vi "Periodic Tasks.vi"(8 "error in":errorcluster, 11 "Begin Cluster":T2={"Left Drive Encoder"={"DevStatus"={"status"=FALSE, "code"=0, "source"=""}, "EncoderIndex"=enum."Enc 0", "CounterIndex"=enum."Invalid", "DistancePerCount"=1.0, "Decoding Type"=enum."4x"}, "Right Drive Encoder"={"DevStatus"={"status"=FALSE, "code"=0, "source"=""}, "EncoderIndex"=enum."Enc 1", "CounterIndex"=enum."Invalid", "DistancePerCount"=1.0, "Decoding Type"=enum."4x"}, "Elevator Encoder"={"DevStatus"={"status"=FALSE, "code"=0, "source"=""}, "EncoderIndex"=enum."Enc 2", "CounterIndex"=enum."Invalid", "DistancePerCount"=1.0, "Decoding Type"=enum."4x"}, "Drive Shifter"={"DevStatus"={"status"=FALSE, "code"=0, "source"=""}, "Pneumatics Control Module"=0, "Forward Solenoid Channel"=enum."Solenoid 0", "Reverse Solenoid Channel"=enum."Solenoid 1"}, "Elevator Shifter"={"DevStatus"={"status"=FALSE, "code"=0, "source"=""}, "Pneumatics Control Module"=0, "Forward Solenoid Channel"=enum."Solenoid 2", "Reverse Solenoid Channel"=enum."Solenoid 3"}, "Elevator Brake"={"DevStatus"={"status"=FALSE, "code"=0, "source"=""}, "Pneumatics Control Module"=0, "Forward Solenoid Channel"=enum."Solenoid 4", "Reverse Solenoid Channel"=enum."Solenoid 5"}, "Intake Clamp"={"DevStatus"={"status"=FALSE, "code"=0, "source"=""}, "Pneumatics Control Module"=0, "Forward Solenoid Channel"=enum."Invalid", "Reverse Solenoid Channel"=enum."Invalid"}, "Intake Hinge"={"DevStatus"={"status"=FALSE, "code"=0, "source"=""}, "Pneumatics Control Module"=0, "Forward Solenoid Channel"=enum."Invalid", "Reverse Solenoid Channel"=enum."Invalid"}, "Pot Left"={"DevStatus"={"status"=FALSE, "code"=0, "source"=""}, "Analog Channel"=enum."AI 0", "Invert Output"=FALSE}, "Pot Right"={"DevStatus"={"status"=FALSE, "code"=0, "source"=""}, "Analog Channel"=enum."AI 1", "Invert Output"=FALSE}, "Gyro"={"DevStatus"={"status"=FALSE, "code"=0, "source"=""}, "Analog Channel"=enum."AI 1", "Gain (VoltsPerDegree/Second)"=0.0, "Gyro Type"=enum."XRS450", "Handle"=8, "SPI Bus"=enum."SPI On-Board, CS0", "Device Found"=TRUE, "Sample Rate"=2000.0, "Calibrate On Open"=FALSE, "Offset"=0.849940624999998}, "Drive Motors"={"DevStatus"={"status"=FALSE, "code"=0, "source"=""}, "Motors[]"=[{"DeviceStatus"={"status"=FALSE, "code"=0, "source"=""}, "Type"=enum."CAN", "PWM"={"PWM Channel"=enum."PWM 1", "DeadBand"={"Name"="", "maxPositivePwm"=0, "minPositivePwm"=0, "centerPwm"=0, "maxNegativePwm"=0, "minNegativePwm"=0, "angularRange"=0}}, "CAN"={"Device Number"=1, "SetOutput VI Ref"=variant(refnum<vi> refnum), "GetOutput VI Ref"=variant(refnum<vi> refnum), "Enable VI Ref"=variant(refnum<vi> refnum), "Disable VI Ref"=variant(refnum<vi> refnum), "Data"=variant(cluster{"Library":path, "handle":u64, "Control Mode":u16, "UsageFrame":u32, "RefNumName":string, "arbID":u32} {"Library"=path "libCTRE_PhoenixCCI.so", "handle"=38411456, "Control Mode"=0, "UsageFrame"=0, "RefNumName"="", "arbID"=33816577})}, "Invert"=TRUE, "DIO PWM"={"PWM \"Enable\" Channel"=enum."Invalid", "DIOChannel"=enum."Invalid", "PWM Rate"=0.0}}, {"DeviceStatus"={"status"=FALSE, "code"=0, "source"=""}, "Type"=enum."CAN", "PWM"={"PWM Channel"=enum."PWM 1", "DeadBand"={"Name"="", "maxPositivePwm"=0, "minPositivePwm"=0, "centerPwm"=0, "maxNegativePwm"=0, "minNegativePwm"=0, "angularRange"=0}}, "CAN"={"Device Number"=13, "SetOutput VI Ref"=variant(refnum<vi> refnum), "GetOutput VI Ref"=variant(refnum<vi> refnum), "Enable VI Ref"=variant(refnum<vi> refnum), "Disable VI Ref"=variant(refnum<vi> refnum), "Data"=variant(cluster{"Library":path, "handle":u64, "Control Mode":u16, "UsageFrame":u32, "RefNumName":string, "arbID":u32} {"Library"=path "libCTRE_PhoenixCCI.so", "handle"=38441312, "Control Mode"=0, "UsageFrame"=0, "RefNumName"="", "arbID"=33816589})}, "Invert"=FALSE, "DIO PWM"={"PWM \"Enable\" Channel"=enum."Invalid", "DIOChannel"=enum."Invalid", "PWM Rate"=0.0}}], "Square Inputs"=FALSE, "Max Output"=1.0}, "Elevator Master"={"DeviceStatus"={"status"=FALSE, "code"=0, "source"=""}, "Type"=enum."CAN", "PWM"={"PWM Channel"=enum."PWM 1", "DeadBand"={"Name"="", "maxPositivePwm"=0, "minPositivePwm"=0, "centerPwm"=0, "maxNegativePwm"=0, "minNegativePwm"=0, "angularRange"=0}}, "CAN"={"Device Number"=9, "SetOutput VI Ref"=variant(refnum<vi> refnum), "GetOutput VI Ref"=variant(refnum<vi> refnum), "Enable VI Ref"=variant(refnum<vi> refnum), "Disable VI Ref"=variant(refnum<vi> refnum), "Data"=variant(cluster{"Library":path, "handle":u64, "Control Mode":u16, "UsageFrame":u32, "RefNumName":string, "arbID":u32} {"Library"=path "libCTRE_PhoenixCCI.so", "handle"=38410640, "Control Mode"=0, "UsageFrame"=0, "RefNumName"="", "arbID"=33816585})}, "Invert"=TRUE, "DIO PWM"={"PWM \"Enable\" Channel"=enum."Invalid", "DIOChannel"=enum."Invalid", "PWM Rate"=0.0}}, "Intake Left"={"DeviceStatus"={"status"=FALSE, "code"=0, "source"=""}, "Type"=enum."CAN", "PWM"={"PWM Channel"=enum."PWM 1", "DeadBand"={"Name"="", "maxPositivePwm"=0, "minPositivePwm"=0, "centerPwm"=0, "maxNegativePwm"=0, "minNegativePwm"=0, "angularRange"=0}}, "CAN"={"Device Number"=6, "SetOutput VI Ref"=variant(refnum<vi> refnum), "GetOutput VI Ref"=variant(refnum<vi> refnum), "Enable VI Ref"=variant(refnum<vi> refnum), "Disable VI Ref"=variant(refnum<vi> refnum), "Data"=variant(cluster{"Library":path, "handle":u64, "Control Mode":u16, "UsageFrame":u32, "RefNumName":string, "arbID":u32} {"Library"=path "libCTRE_PhoenixCCI.so", "handle"=38393360, "Control Mode"=0, "UsageFrame"=0, "RefNumName"="", "arbID"=33816582})}, "Invert"=FALSE, "DIO PWM"={"PWM \"Enable\" Channel"=enum."Invalid", "DIOChannel"=enum."Invalid", "PWM Rate"=0.0}}, "Intake Right"={"DeviceStatus"={"status"=FALSE, "code"=0, "source"=""}, "Type"=enum."CAN", "PWM"={"PWM Channel"=enum."PWM 1", "DeadBand"={"Name"="", "maxPositivePwm"=0, "minPositivePwm"=0, "centerPwm"=0, "maxNegativePwm"=0, "minNegativePwm"=0, "angularRange"=0}}, "CAN"={"Device Number"=7, "SetOutput VI Ref"=variant(refnum<vi> refnum), "GetOutput VI Ref"=variant(refnum<vi> refnum), "Enable VI Ref"=variant(refnum<vi> refnum), "Disable VI Ref"=variant(refnum<vi> refnum), "Data"=variant(cluster{"Library":path, "handle":u64, "Control Mode":u16, "UsageFrame":u32, "RefNumName":string, "arbID":u32} {"Library"=path "libCTRE_PhoenixCCI.so", "handle"=38392544, "Control Mode"=0, "UsageFrame"=0, "RefNumName"="", "arbID"=33816583})}, "Invert"=FALSE, "DIO PWM"={"PWM \"Enable\" Channel"=enum."Invalid", "DIOChannel"=enum."Invalid", "PWM Rate"=0.0}}, "Linear Actuator Left"={"DeviceStatus"={"status"=FALSE, "code"=0, "source"=""}, "Type"=enum."CAN", "PWM"={"PWM Channel"=enum."PWM 1", "DeadBand"={"Name"="", "maxPositivePwm"=0, "minPositivePwm"=0, "centerPwm"=0, "maxNegativePwm"=0, "minNegativePwm"=0, "angularRange"=0}}, "CAN"={"Device Number"=4, "SetOutput VI Ref"=variant(refnum<vi> refnum), "GetOutput VI Ref"=variant(refnum<vi> refnum), "Enable VI Ref"=variant(refnum<vi> refnum), "Disable VI Ref"=variant(refnum<vi> refnum), "Data"=variant(cluster{"Library":path, "handle":u64, "Control Mode":u16, "UsageFrame":u32, "RefNumName":string, "arbID":u32} {"Library"=path "libCTRE_PhoenixCCI.so", "handle"=36427792, "Control Mode"=0, "UsageFrame"=0, "RefNumName"="", "arbID"=33816580})}, "Invert"=FALSE, "DIO PWM"={"PWM \"Enable\" Channel"=enum."Invalid", "DIOChannel"=enum."Invalid", "PWM Rate"=0.0}}, "Linear Actuator Right"={"DeviceStatus"={"status"=FALSE, "code"=0, "source"=""}, "Type"=enum."CAN", "PWM"={"PWM Channel"=enum."PWM 1", "DeadBand"={"Name"="", "maxPositivePwm"=0, "minPositivePwm"=0, "centerPwm"=0, "maxNegativePwm"=0, "minNegativePwm"=0, "angularRange"=0}}, "CAN"={"Device Number"=5, "SetOutput VI Ref"=variant(refnum<vi> refnum), "GetOutput VI Ref"=variant(refnum<vi> refnum), "Enable VI Ref"=variant(refnum<vi> refnum), "Disable VI Ref"=variant(refnum<vi> refnum), "Data"=variant(cluster{"Library":path, "handle":u64, "Control Mode":u16, "UsageFrame":u32, "RefNumName":string, "arbID":u32} {"Library"=path "libCTRE_PhoenixCCI.so", "handle"=38440496, "Control Mode"=0, "UsageFrame"=0, "RefNumName"="", "arbID"=33816581})}, "Invert"=FALSE, "DIO PWM"={"PWM \"Enable\" Channel"=enum."Invalid", "DIOChannel"=enum."Invalid", "PWM Rate"=0.0}}, "X Joystick"={"Device"=enum."USB 0"}, "Y Joystick"={"Device"=enum."USB 1"}, "Controller"={"Device"=enum."USB 2"}, "775 Drive Motors"={"DevStatus"={"status"=FALSE, "code"=0, "source"=""}, "Motors[]"=[{"DeviceStatus"={"status"=FALSE, "code"=0, "source"=""}, "Type"=enum."CAN", "PWM"={"PWM Channel"=enum."PWM 1", "DeadBand"={"Name"="", "maxPositivePwm"=0, "minPositivePwm"=0, "centerPwm"=0, "maxNegativePwm"=0, "minNegativePwm"=0, "angularRange"=0}}, "CAN"={"Device Number"=3, "SetOutput VI Ref"=variant(refnum<vi> refnum), "GetOutput VI Ref"=variant(refnum<vi> refnum), "Enable VI Ref"=variant(refnum<vi> refnum), "Disable VI Ref"=variant(refnum<vi> refnum), "Data"=variant(cluster{"Library":path, "handle":u64, "Control Mode":u16, "UsageFrame":u32, "RefNumName":string, "arbID":u32} {"Library"=path "libCTRE_PhoenixCCI.so", "handle"=38456632, "Control Mode"=0, "UsageFrame"=0, "RefNumName"="", "arbID"=33816579})}, "Invert"=FALSE, "DIO PWM"={"PWM \"Enable\" Channel"=enum."Invalid", "DIOChannel"=enum."Invalid", "PWM Rate"=0.0}}, {"DeviceStatus"={"status"=FALSE, "code"=0, "source"=""}, "Type"=enum."CAN", "PWM"={"PWM Channel"=enum."PWM 1", "DeadBand"={"Name"="", "maxPositivePwm"=0, "minPositivePwm"=0, "centerPwm"=0, "maxNegativePwm"=0, "minNegativePwm"=0, "angularRange"=0}}, "CAN"={"Device Number"=11, "SetOutput VI Ref"=variant(refnum<vi> refnum), "GetOutput VI Ref"=variant(refnum<vi> refnum), "Enable VI Ref"=variant(refnum<vi> refnum), "Disable VI Ref"=variant(refnum<vi> refnum), "Data"=variant(cluster{"Library":path, "handle":u64, "Control Mode":u16, "UsageFrame":u32, "RefNumName":string, "arbID":u32} {"Library"=path "libCTRE_PhoenixCCI.so", "handle"=36428608, "Control Mode"=0, "UsageFrame"=0, "RefNumName"="", "arbID"=33816587})}, "Invert"=TRUE, "DIO PWM"={"PWM \"Enable\" Channel"=enum."Invalid", "DIOChannel"=enum."Invalid", "PWM Rate"=0.0}}], "Square Inputs"=FALSE, "Max Output"=1.0}, "Intake Angle Encoder"={"DevStatus"={"status"=FALSE, "code"=0, "source"=""}, "EncoderIndex"=enum."Enc 3", "CounterIndex"=enum."Invalid", "DistancePerCount"=1.0, "Decoding Type"=enum."4x"}, "Intake Angle"={"DeviceStatus"={"status"=FALSE, "code"=0, "source"=""}, "Type"=enum."CAN", "PWM"={"PWM Channel"=enum."PWM 1", "DeadBand"={"Name"="", "maxPositivePwm"=0, "minPositivePwm"=0, "centerPwm"=0, "maxNegativePwm"=0, "minNegativePwm"=0, "angularRange"=0}}, "CAN"={"Device Number"=8, "SetOutput VI Ref"=variant(refnum<vi> refnum), "GetOutput VI Ref"=variant(refnum<vi> refnum), "Enable VI Ref"=variant(refnum<vi> refnum), "Disable VI Ref"=variant(refnum<vi> refnum), "Data"=variant(cluster{"Library":path, "handle":u64, "Control Mode":u16, "UsageFrame":u32, "RefNumName":string, "arbID":u32} {"Library"=path "libCTRE_PhoenixCCI.so", "handle"=38391728, "Control Mode"=0, "UsageFrame"=0, "RefNumName"="", "arbID"=33816584})}, "Invert"=FALSE, "DIO PWM"={"PWM \"Enable\" Channel"=enum."Invalid", "DIOChannel"=enum."Invalid", "PWM Rate"=0.0}}} {"Gyro"."Sample Rate" min=0.25 max=100.0 step=0.25}) -> ()   [LabVIEW 2017]
doc: "This VI runs in parallel to other tasks. It can contain as many user-defined periodic loops as you need. These can carry out PID or other sorts of timed response."
uses:
  Begin Cluster.ctl
  <vilib>/Rock Robotics/WPI/Encoder/WPI_EncoderDevRef.ctl
  <vilib>/Rock Robotics/SystemInterfaces/Encoder/FPGA_EncoderIdx.ctl
  <vilib>/Rock Robotics/SystemInterfaces/Counter/FPGA_CounterCtrSystemIndex.ctl
  <vilib>/Rock Robotics/WPI/Encoder/WPI_EncoderType.ctl
  <vilib>/Rock Robotics/WPI/Solenoid/WPI_SolenoidDevRef.ctl
  <vilib>/Rock Robotics/WPI/Solenoid/WPI_SolenoidChannel.ctl
  <vilib>/Rock Robotics/WPI/Potentiometer/WPI_PotentiometerDevRef.ctl
  <vilib>/Rock Robotics/SystemInterfaces/AI/FPGA_AIChannel.ctl
  <vilib>/Rock Robotics/WPI/Gyro/WPI_GyroDevRef.ctl
  <vilib>/Rock Robotics/SystemInterfaces/spilib/spi_bus.ctl
  <vilib>/Rock Robotics/WPI/RobotDrive/WPI_RobotDriveDevRef.ctl
  <vilib>/Rock Robotics/WPI/MotorControl/WPI_MotorControlDeviceRef.ctl
  <vilib>/Rock Robotics/WPI/MotorControl/WPI_MotorControlType.ctl
  <vilib>/Rock Robotics/SystemInterfaces/DIO/FPGA_DIOPWMChannel.ctl
  <vilib>/Rock Robotics/WPI/PWM/WPI_PWMDeadband.ctl
  <vilib>/Rock Robotics/SystemInterfaces/DIO/FPGA_DIOChannel.ctl
  <vilib>/Rock Robotics/WPI/Joystick/WPI_JoystickDevRef.ctl
  <vilib>/Rock Robotics/WPI/Joystick/WPI_JoystickDeviceEnum.ctl
  <vilib>/Rock Robotics/WPI/Solenoid/WPI_SolenoidValue.ctl
  Global Variables.vi
  <vilib>/addons/control/pid/pid.llb/PID (DBL).vi
  <vilib>/Rock Robotics/WPI/Solenoid/WPI_SolenoidSetEnum.vi
  <vilib>/Rock Robotics/Network Tables/NT Read Number.vi
  <vilib>/Rock Robotics/Network Tables/NT Write Boolean.vi
  <vilib>/addons/control/pid/NI_PID_pid.lvlib
panel:
  out "Intake Encoder":dbl
  out "Right Encoder":dbl
  out "Side":dbl
  out "Field option":dbl
  out "Elevator Topped Out":bool
  in  "Intake PID Gains":T1={"proportional gain (Kc)"=0.06610000000000005, "integral time (Ti, min)"=0.0, "derivative time (Td, min)"=0.002} {"derivative time (Td, min)" format="%.3f"; "integral time (Ti, min)" format="%.3f"; "proportional gain (Kc)" format="%.3f"}
  in  "Intake Range":cluster{"output high":dbl, "output low":dbl}={"output high"=1.0, "output low"=-1.0} {"output low" format="%.2f"; "output high" format="%.2f"}
  in  "Elevator Gains High":T1={"proportional gain (Kc)"=0.0008, "integral time (Ti, min)"=0.0, "derivative time (Td, min)"=0.0} {"proportional gain (Kc)" format="%#_7g"}
  out "Elevator Encoder":dbl=-256.25
  out "Normalized Value":dbl=0.6625300700982322
  in  "Elevator Gains Low":T1={"proportional gain (Kc)"=0.0011, "integral time (Ti, min)"=0.0, "derivative time (Td, min)"=0.0} {"derivative time (Td, min)" format="%.3f"; "integral time (Ti, min)" format="%.3f"; "proportional gain (Kc)" format="%.5f"}
  in  "Cube Up":bool
  in  "Cube Down":bool
  out "Angle":dbl=-3.1437039937493667
  out "Left Encoder":dbl=-0.5
  # "Analog"
  # "XRS"
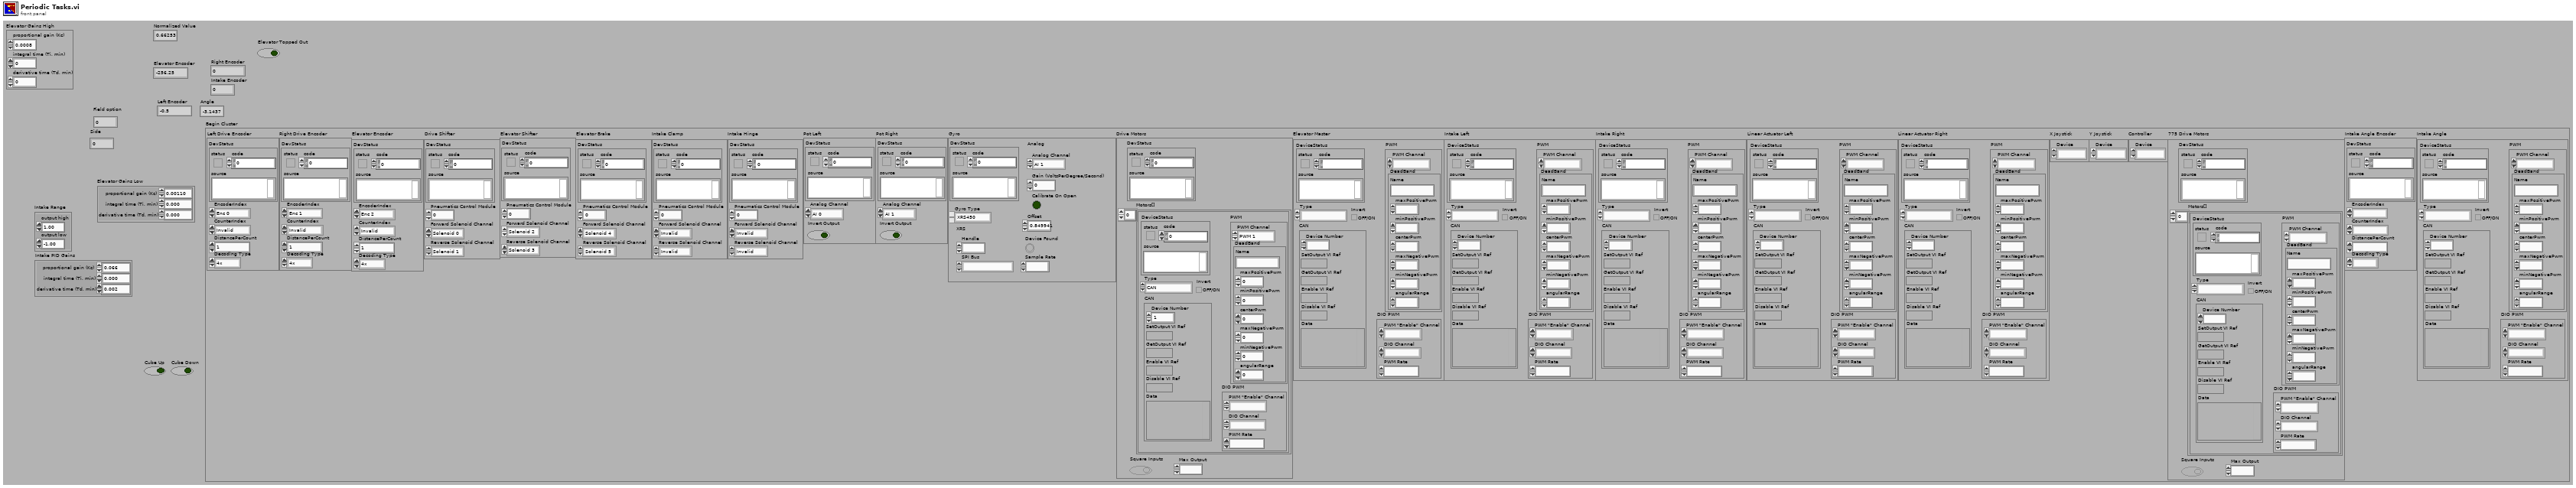
[diagram p1: front panel]
types:
  T1 = cluster{"proportional gain (Kc)":dbl, "integral time (Ti, min)":dbl, "derivative time (Td, min)":dbl}
  T2 = typedef "Begin Cluster.ctl" = cluster{"Left Drive Encoder":T3, "Right Drive Encoder":T3, "Elevator Encoder":T3, "Drive Shifter":T7, "Elevator Shifter":T7, "Elevator Brake":T7, "Intake Clamp":T7, "Intake Hinge":T7, "Pot Left":T9, "Pot Right":T9, "Gyro":T11, "Drive Motors":T13, "Elevator Master":T14, "Intake Left":T14, "Intake Right":T14, "Linear Actuator Left":T14, "Linear Actuator Right":T14, "X Joystick":T19, "Y Joystick":T19, "Controller":T19, "775 Drive Motors":T13, "Intake Angle Encoder":T3, "Intake Angle":T14}
  T3 = typedef "WPI_EncoderDevRef.ctl" = cluster{"DevStatus":errorcluster, "EncoderIndex":T4, "CounterIndex":T5, "DistancePerCount":dbl, "Decoding Type":T6}
  T4 = typedef "FPGA_EncoderIdx.ctl" = enum8{"Enc 0", "Enc 1", "Enc 2", "Enc 3", "Enc 4", "Enc 5", "Enc 6", "Enc 7", "Invalid"}
  T5 = typedef "FPGA_CounterCtrSystemIndex.ctl" = enum8{"Ctr 0", "Ctr 1", "Ctr 2", "Ctr 3", "Ctr 4", "Ctr 5", "Ctr 6", "Ctr 7", "Invalid"}
  T6 = typedef "WPI_EncoderType.ctl" = enum16{"1x", "2x", "4x"}
  T7 = typedef "WPI_SolenoidDevRef.ctl" = cluster{"DevStatus":errorcluster, "Pneumatics Control Module":u8, "Forward Solenoid Channel":T8, "Reverse Solenoid Channel":T8}
  T8 = typedef "WPI_SolenoidChannel.ctl" = enum8{"Solenoid 0", "Solenoid 1", "Solenoid 2", "Solenoid 3", "Solenoid 4", "Solenoid 5", "Solenoid 6", "Solenoid 7", "Invalid"}
  T9 = typedef "WPI_PotentiometerDevRef.ctl" = cluster{"DevStatus":errorcluster, "Analog Channel":T10, "Invert Output":bool}
  T10 = typedef "FPGA_AIChannel.ctl" = enum8{"AI 0", "AI 1", "AI 2", "AI 3", "AI MXP 0", "AI MXP 1", "AI MXP 2", "AI MXP 3", "Invalid"}
  T11 = typedef "WPI_GyroDevRef.ctl" = cluster{"DevStatus":errorcluster, "Analog Channel":T10, "Gain (VoltsPerDegree/Second)":dbl, "Gyro Type":enum16{"Analog", "XRS450"}, "Handle":i32, "SPI Bus":T12, "Device Found":bool, "Sample Rate":dbl, "Calibrate On Open":bool, "Offset":dbl}
  T12 = typedef "spi_bus.ctl" = enum16{"SPI On-Board, CS0", "SPI On-Board, CS1", "SPI On-Board, CS2", "SPI On-Board, CS3", "SPI MXP", "Invalid"}
  T13 = typedef "WPI_RobotDriveDevRef.ctl" = cluster{"DevStatus":errorcluster, "Motors[]":T14[], "Square Inputs":bool, "Max Output":dbl}
  T14 = typedef "WPI_MotorControlDeviceRef.ctl" = cluster{"DeviceStatus":errorcluster, "Type":T15, "PWM":cluster{"PWM Channel":T16, "DeadBand":T17}, "CAN":cluster{"Device Number":u8, "SetOutput VI Ref":variant, "GetOutput VI Ref":variant, "Enable VI Ref":variant, "Disable VI Ref":variant, "Data":variant}, "Invert":bool, "DIO PWM":cluster{"PWM \"Enable\" Channel":T16, "DIOChannel":T18, "PWM Rate":dbl}}
  T15 = typedef "WPI_MotorControlType.ctl" = enum16{"PWM", "CAN", "DIO PWM"}
  T16 = typedef "FPGA_DIOPWMChannel.ctl" = enum8{"PWM 0", "PWM 1", "PWM 2", "PWM 3", "PWM 4", "PWM 5", "PWM 6", "PWM 7", "PWM 8", "PWM 9", "PWM MXP 0", "PWM MXP 1", "PWM MXP 2", "PWM MXP 3", "PWM MXP 4", "PWM MXP 5", "PWM MXP 6", "PWM MXP 7", "PWM MXP 8", "PWM MXP 9", "Invalid"}
  T17 = typedef "WPI_PWMDeadband.ctl" = cluster{"Name":string, "maxPositivePwm":i32, "minPositivePwm":i32, "centerPwm":i32, "maxNegativePwm":i32, "minNegativePwm":i32, "angularRange":u16}
  T18 = typedef "FPGA_DIOChannel.ctl" = enum8{"DIO 0", "DIO 1", "DIO 2", "DIO 3", "DIO 4", "DIO 5", "DIO 6", "DIO 7", "DIO 8", "DIO 9", "DIO MXP 0", "DIO MXP 1", "DIO MXP 2", "DIO MXP 3", "DIO MXP 4", "DIO MXP 5", "DIO MXP 6", "DIO MXP 7", "DIO MXP 8", "DIO MXP 9", "DIO MXP 10", "DIO MXP 11", "DIO MXP 12", "DIO MXP 13", "DIO MXP 14", "DIO MXP 15", "SPI Port CS1", "SPI Port CS2", "SPI Port CS3", "SPI Port MISO", "SPI Port MOSI", "Invalid"}
  T19 = typedef "WPI_JoystickDevRef.ctl" = cluster{"Device":T20}
  T20 = typedef "WPI_JoystickDeviceEnum.ctl" = enum16{"USB 0", "USB 1", "USB 2", "USB 3", "USB 4", "USB 5"}
  T21 = typedef "WPI_SolenoidValue.ctl" = enum16{"Off", "On", "Forward", "Reverse"}
  T22 = typedef "GRIP Contours Report.ctl" = cluster{"area":dbl, "centerX":dbl, "centerY":dbl, "width":dbl, "height":dbl, "solidity":dbl}
  T23 = enum16{"Idle", "Ground", "Portal", "Switch", "Scale", "Cube Down", "Cube Up", "Add Down", "Add Up"}
  T24 = enum16{"Idle", "Portal", "Subtract", "Add", "Straight Up"}
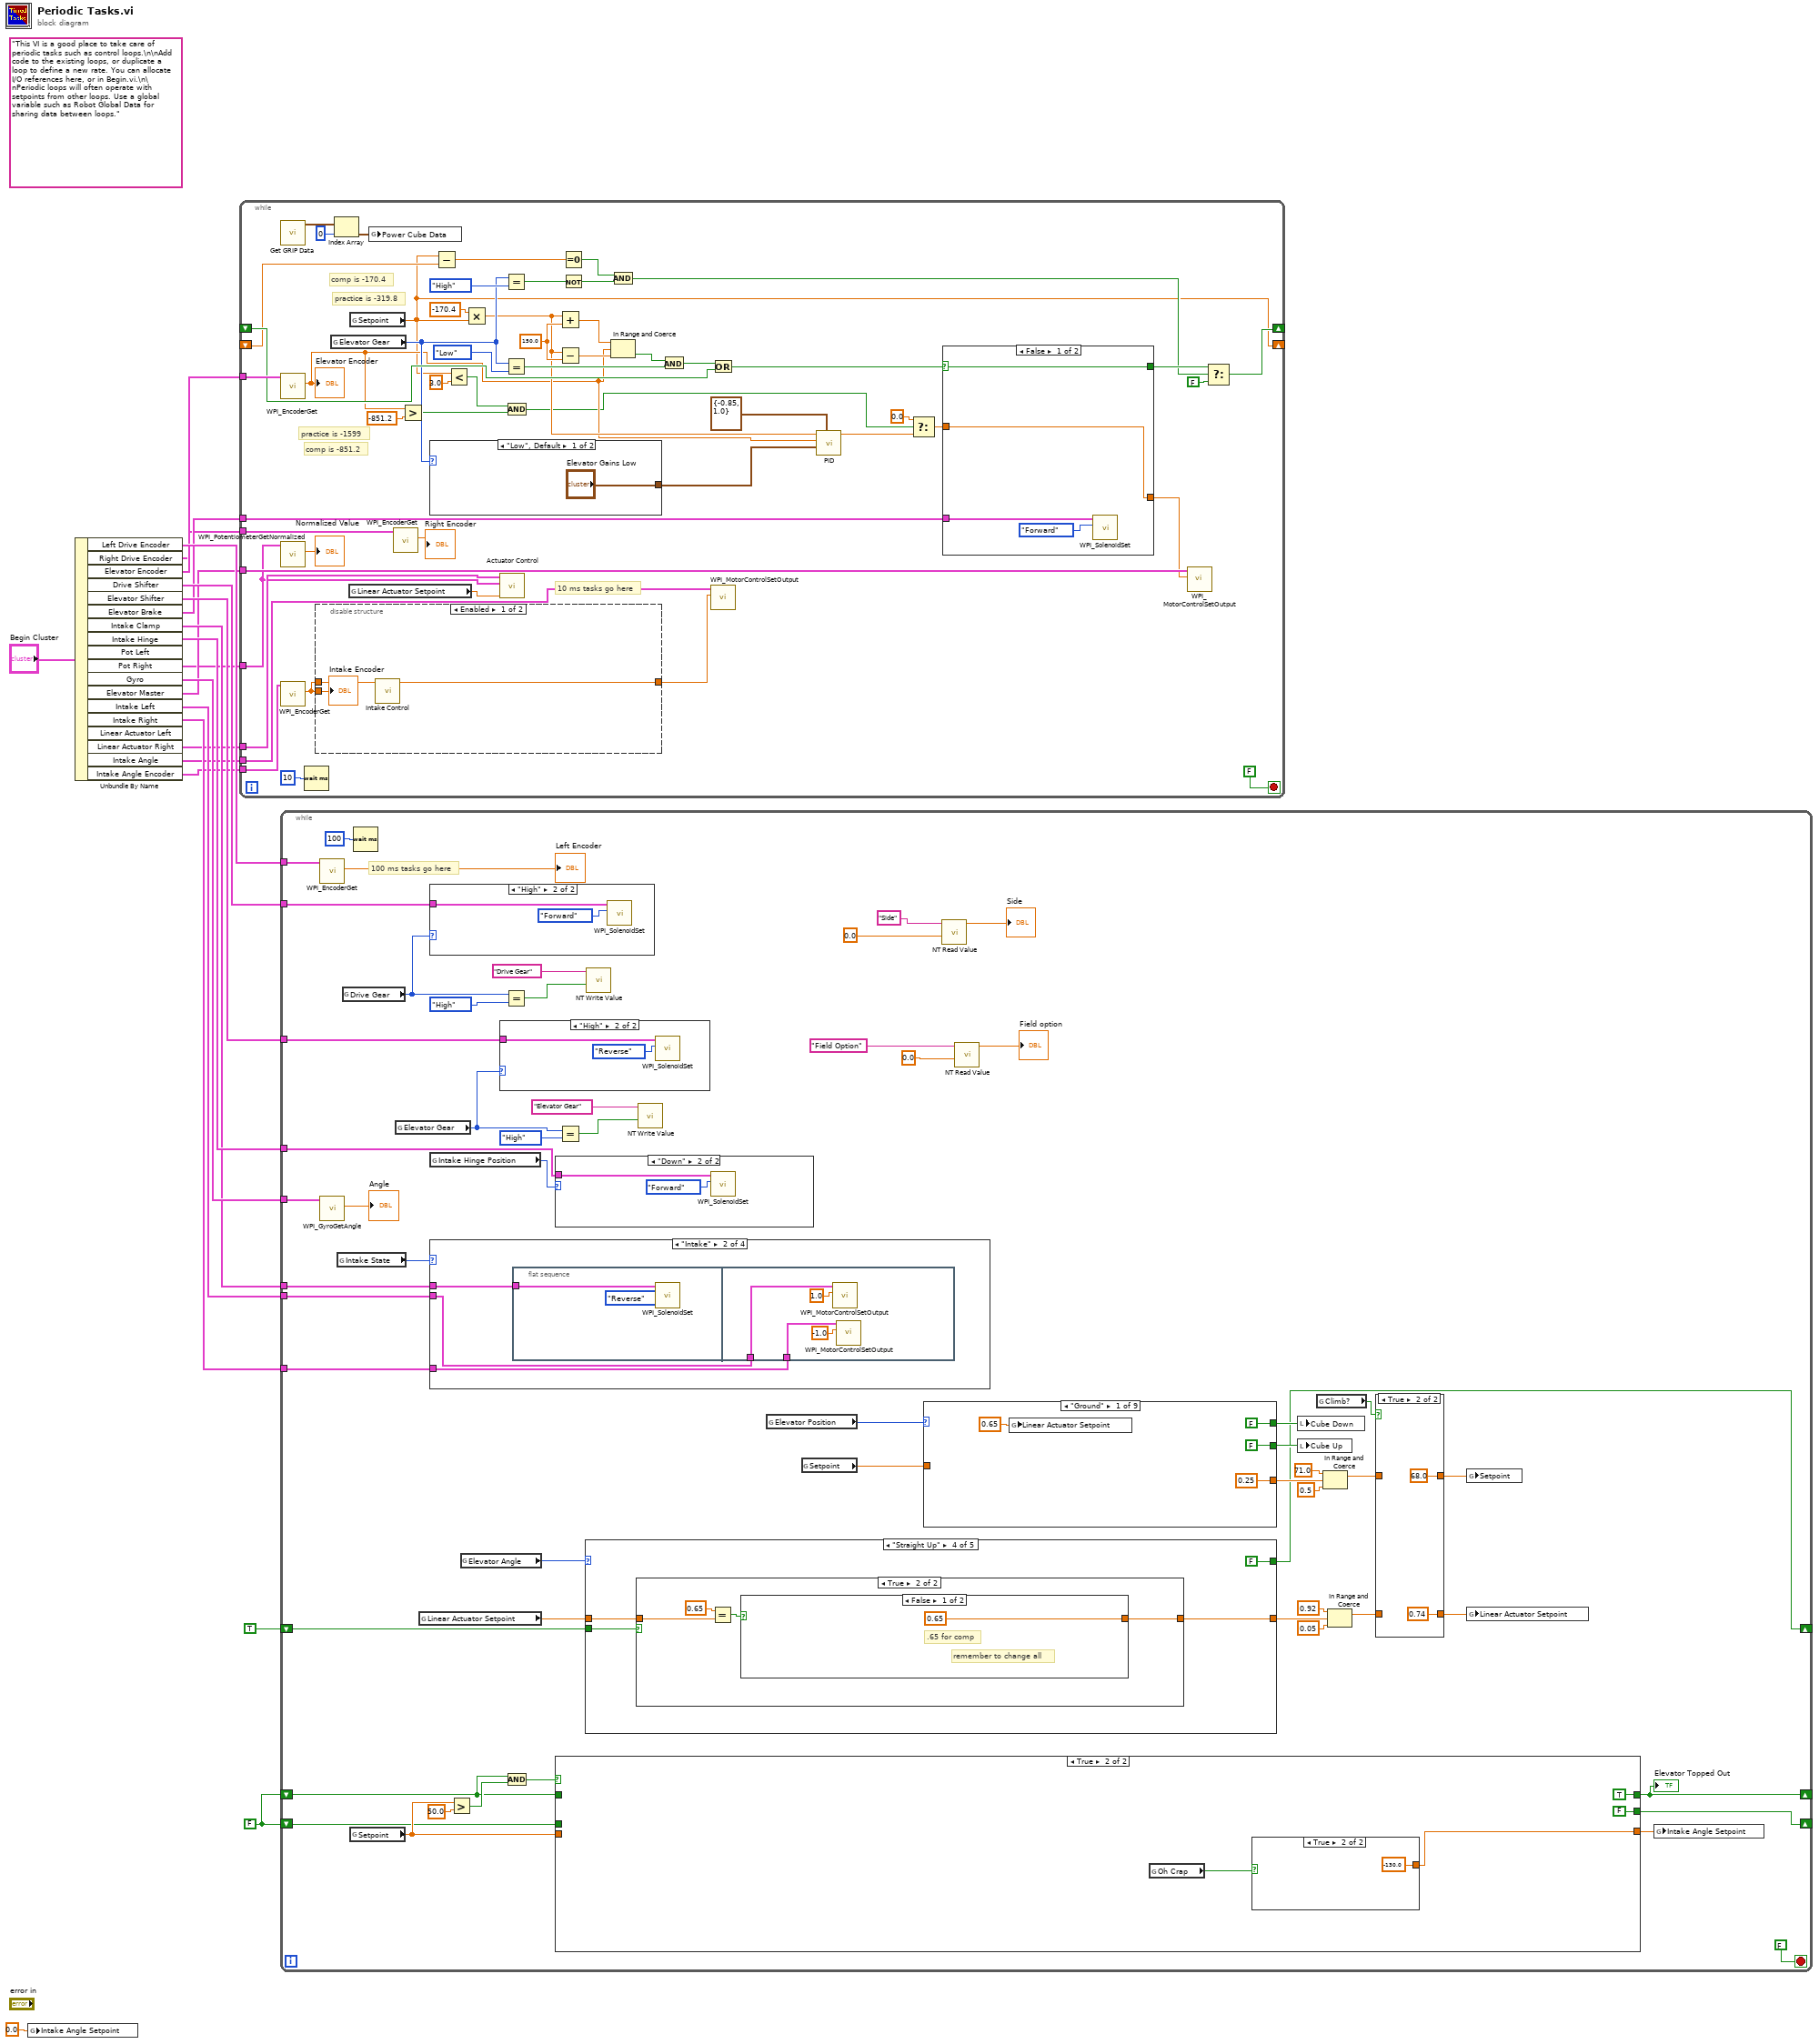
[diagram p0: block diagram]
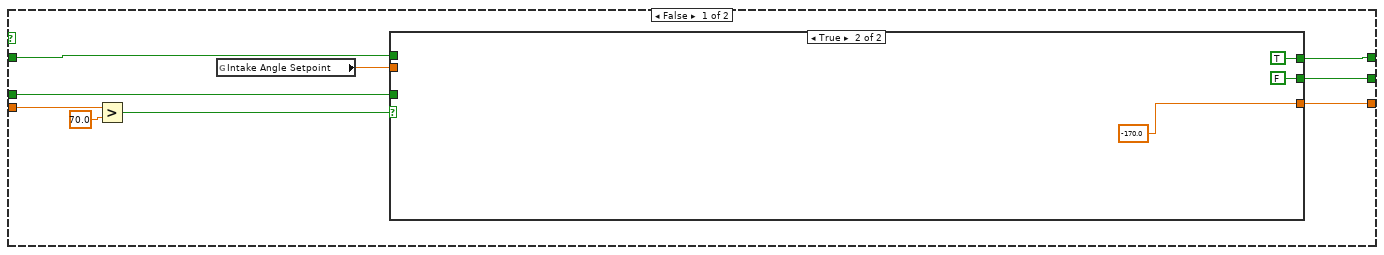
[diagram p2: hidden frame]
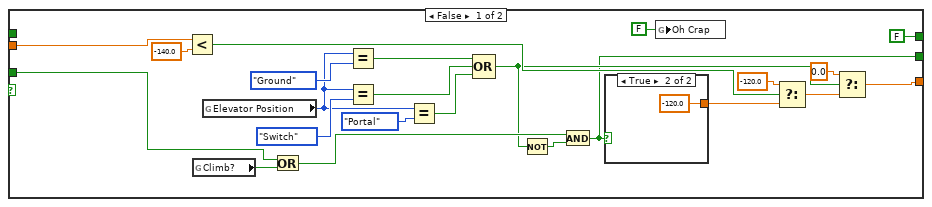
[diagram p3: hidden frame]
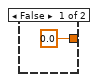
[diagram p4: hidden frame]
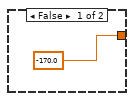
[diagram p5: hidden frame]
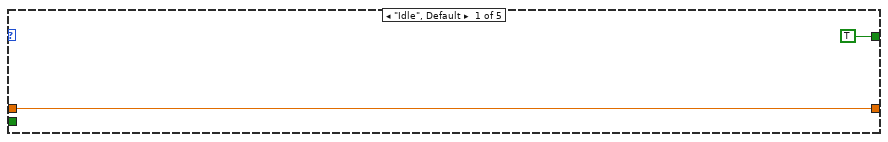
[diagram p7: hidden frame]
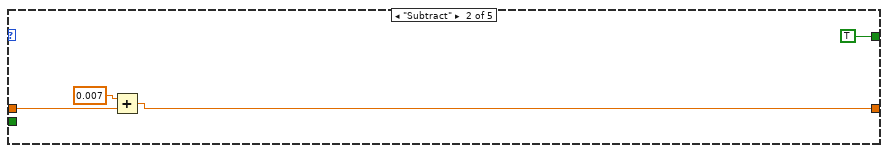
[diagram p8: hidden frame]
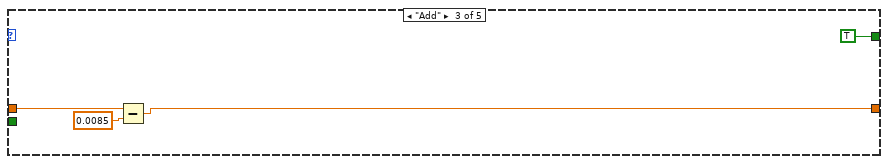
[diagram p9: hidden frame]
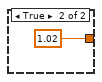
[diagram p11: hidden frame]
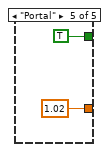
[diagram p12: hidden frame]
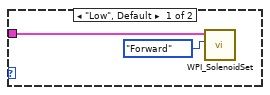
[diagram p13: hidden frame]
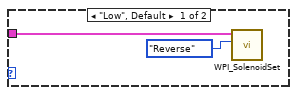
[diagram p14: hidden frame]
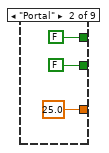
[diagram p15: hidden frame]
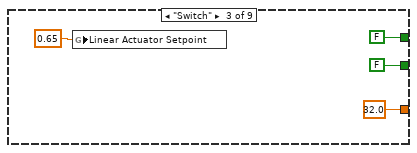
[diagram p16: hidden frame]
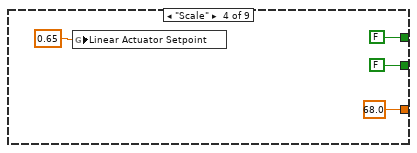
[diagram p17: hidden frame]
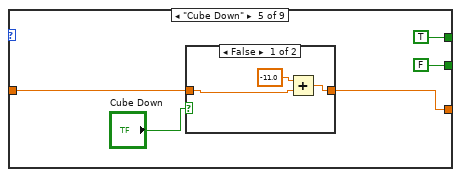
[diagram p18: hidden frame]
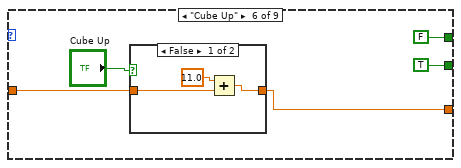
[diagram p20: hidden frame]
diagram:
  w2 = FALSE
  (unwired) "This VI is a good place to take care of periodic tasks such as control loops.\n\nAdd code to the existing loops, or duplicate a loop to define a new rate. You can allocate I/O references here, or in Begin.vi.\n\nPeriodic loops will often operate with setpoints from other loops. Use a global variable such as Robot Global Data for sharing data between loops."
  n1 = global write "Global Variables.vi" "Intake Angle Setpoint"(0.0 ("Intake Angle Setpoint")) -> ()
  n2 = Unbundle By Name("Begin Cluster") -> ("Left Drive Encoder"=w19:T3, "Right Drive Encoder"=w1:T3, "Elevator Encoder"=w7:T3, "Drive Shifter"=w12:T7, "Elevator Shifter"=w13:T7, "Elevator Brake"=w8:T7, "Intake Clamp"=w14:T7, "Intake Hinge"=w15:T7, "Pot Right"=w9:T9, "Gyro"=w16:T11, "Elevator Master"=w11:T14, "Intake Left"=w18:T14, "Intake Right"=w17:T14, "Linear Actuator Right"=w10:T14, "Intake Angle"=w4:T14, "Intake Angle Encoder"=w5:T3)  [unwired: 2 out]
  n3 = while {
    tunnel: w11 -> [w67]
    tunnel: w10 -> [w36]
    tunnel: w9 -> [w34]
    tunnel: w8 -> [w66]
    tunnel: w7 -> [w65]
    tunnel: w5 -> [w60]
    tunnel: w4 -> [w59]
    shift-right: [w46] -> _
    shift-left: _ -> [w51]
    shift-right: [w27] -> _
    shift-left: _ -> [w49]
    tunnel: w1 -> [w22]
    stop <- FALSE stop-if-true
    w63 = 150.0 ("y")
    # "comp is -851.2"
    # "comp is -170.4"
    # "practice is -1599"
    # "practice is -319.8"
    # "10 ms tasks go here"
    n4 = call "Get GRIP Data.vi"() -> ("ContoursReport"=w71:T22[])  [unwired: 9 in, 2 out]
    n5 = call <vilib>:"WPI_EncoderGet.vi"("EncoderDevRef"=w65) -> ("Distance"=w28:dbl)  [unwired: 5 in, 5 out]
    "Elevator Encoder" <- w28
    n6 = call <vilib>:"WPI_PotentiometerGetNormalized.vi"("PotDevRef"=w34) -> ("Normalized Value"=→"Normalized Value":dbl)  [unwired: 8 in, 2 out]
    n7 = call <vilib>:"WPI_EncoderGet.vi"("EncoderDevRef"=w60) -> ("Distance"=w44:dbl)  [unwired: 5 in, 5 out]
    n8 = Wait (ms)(milliseconds to wait=u32 10) -> ()  [unwired: 1 out]
    n9 = disable-structure shown="Enabled" {
      disable-tunnel: w44 -> [w76 _]
      disable-tunnel: [w75 w78] -> w43
      disable-tunnel: w44 -> [w74 w79]
      frame Enabled {
        n10 = call "Intake Control.vi"("Intake Encoder Angle"=w76) -> ("Intake Motor Power"=w75:dbl)  [unwired: 10 in]
        "Intake Encoder" <- w74
      }
      frame Disabled {
        n11 = global read "Global Variables.vi" "Intake Angle Setpoint"() -> (w80:dbl)
        n12 = call-poly <vilib>:"PID.vi"("output range"="Intake Range", "PID gains"="Intake PID Gains", "process variable"=w79, "setpoint"=w80) -> ("output"=w78:dbl)  [unwired: 6 in, 1 out]
      }
    }
    n13 = global read "Global Variables.vi" "Elevator Gear"() -> (w39:enum16{"Low", "High"})
    n14 = Index Array(array=w71, index=0) -> (element=w69:T22)
    n15 = global read "Global Variables.vi" "Linear Actuator Setpoint"() -> (w35:dbl)
    n16 = global read "Global Variables.vi" "Setpoint"() -> (w27:dbl)
    n17 = global write "Global Variables.vi" "Power Cube Data"(w69) -> ()
    n18 = call <vilib>:"WPI_EncoderGet.vi"("EncoderDevRef"=w22) -> ("Distance"=→"Right Encoder":dbl)  [unwired: 5 in, 5 out]
    n19 = Greater?(x=w28, y=-851.2) -> (0:w25:bool)
    n20 = case shown="\"Low\", Default" w39 {
      tunnel: ["Elevator Gains Low" "Elevator Gains High"] -> w61
      frame "Low", Default {
      }
      frame "High" {
      }
    }
    n21 = Subtract(x=w27, y=w49) -> (x-y=w48:dbl)
    n22 = Less?(x=w27, y=3.0) -> (x < y?=w24:bool)
    n23 = Multiply(x=-170.4, y=w27) -> (x*y=w33:dbl)
    n24 = call "Actuator Control.vi"("setpoint"=w35, "Pot Right"=w34, "Actuator Right"=w36) -> ()  [unwired: 9 in]
    n25 = Equal?(x=w39, y=enum16{"Low", "High"}."High") -> (x = y?=w41:bool)
    n26 = Equal?(x=w39, y=enum16{"Low", "High"}."Low") -> (x = y?=w56:bool)
    n27 = And(x=w24, y=w25) -> (x .and. y?=w23:bool)
    n28 = Add(x=w33, y=w63) -> (x+y=w55:dbl)
    n29 = Subtract(x=w33, y=w63) -> (x-y=w54:dbl)
    n30 = Equal To 0?(x=w48) -> (x = 0?=w42:bool)
    n31 = Not(x=w41) -> (.not. x?=w37:bool)
    n32 = And(x=w42, y=w37) -> (x .and. y?=w38:bool)
    n33 = In Range and Coerce(upper limit=w55, x=w28, lower limit=w54) -> (In Range?=w58:bool)  [unwired: 1 out]
    n34 = And(x=w58, y=w56) -> (x .and. y?=w52:bool)
    n35 = Or(x=w52, y=w51) -> (x .or. y?=w50:bool)
    n36 = call <vilib>:"WPI_MotorControlSetOutput.vi"("Output"=w43, "MotorControlDevRef"=w59) -> ()  [unwired: 7 in, 3 out]
    n37 = call-poly <vilib>:"PID.vi"("output range"=cluster{"output low":dbl, "output high":dbl} {"output low"=-0.85, "output high"=1.0}, "PID gains"=w61, "process variable"=w28, "setpoint"=w33) -> ("output"=w30:dbl)  [unwired: 6 in, 1 out]
    n38 = Select(t=0.0, s=w23, f=w30) -> (s? t:f=w29:dbl)
    n39 = case shown="False" w50 {
      selector: w50 -> [w84 w88]
      tunnel: w66 -> [w86 w90]
      tunnel: w29 -> [w85 _]
      tunnel: [w85 0.0 ("output")] -> w53
      tunnel: [w84 w88] -> w45
      frame False {
        n40 = call-poly <vilib>:"WPI_SolenoidSet.vi"("Value"=WPI_SolenoidValue."Forward", "SolenoidDevRef"=w86) -> ()  [unwired: 8 in, 2 out]
      }
      frame True {
        n41 = call-poly <vilib>:"WPI_SolenoidSet.vi"("Value"=WPI_SolenoidValue."Reverse", "SolenoidDevRef"=w90) -> ()  [unwired: 8 in, 2 out]
      }
    }
    n42 = call <vilib>:"WPI_MotorControlSetOutput.vi"("Output"=w53, "MotorControlDevRef"=w67) -> ()  [unwired: 7 in, 3 out]
    n43 = Select(t=w45, s=w38, f=FALSE) -> (s? t:f=w46:bool)
  }
  n44 = while {
    tunnel: w19 -> [w142]
    tunnel: w18 -> [w136]
    tunnel: w17 -> [w137]
    tunnel: w16 -> [w141]
    tunnel: w15 -> [w139]
    tunnel: w14 -> [w138]
    tunnel: w13 -> [w128]
    tunnel: w12 -> [w127]
    shift-right: [w121] -> _
    shift-left: TRUE -> [w122]
    shift-right: [w110] -> _
    shift-left: w2 -> [w109]
    shift-right: [w108] -> _
    shift-left: w2 -> [w107]
    stop <- FALSE stop-if-true
    # "100 ms tasks go here"
    n45 = call <vilib>:"WPI_EncoderGet.vi"("EncoderDevRef"=w142) -> ("Distance"=→"Left Encoder":dbl)  [unwired: 5 in, 5 out]
    n46 = call <vilib>:"WPI_GyroGetAngle.vi"("GyroDevRef"=w141) -> ("Angle"=→"Angle":dbl)  [unwired: 6 in, 4 out]
    n47 = global read "Global Variables.vi" "Intake State"() -> (w143:enum16{"Off", "Intake", "Spit Low", "Spit High"})
    n48 = global read "Global Variables.vi" "Drive Gear"() -> (w106:enum16{"Low", "High"})
    n49 = global read "Global Variables.vi" "Setpoint"() -> (w111:dbl)
    n50 = Wait (ms)(milliseconds to wait=u32 100) -> ()  [unwired: 1 out]
    n51 = global read "Global Variables.vi" "Elevator Gear"() -> (w101:enum16{"Low", "High"})
    n52 = global read "Global Variables.vi" "Linear Actuator Setpoint"() -> (w124:dbl)
    n53 = case shown="\"High\"" w106 {
      tunnel: w127 -> [w222 w225]
      frame "Low", Default {
        n54 = call-poly <vilib>:"WPI_SolenoidSet.vi"("Value"=WPI_SolenoidValue."Reverse", "SolenoidDevRef"=w222) -> ()  [unwired: 8 in, 2 out]
      }
      frame "High" {
        n55 = call-poly <vilib>:"WPI_SolenoidSet.vi"("Value"=WPI_SolenoidValue."Forward", "SolenoidDevRef"=w225) -> ()  [unwired: 8 in, 2 out]
      }
    }
    n56 = global read "Global Variables.vi" "Intake Hinge Position"() -> (w140:enum16{"Up", "Down"})
    n57 = case shown="\"Intake\"" w143 {
      tunnel: w138 -> [w276 w282 w293 w301]
      tunnel: w137 -> [w274 w283 w292 w300]
      tunnel: w136 -> [w275 w284 w291 w302]
      frame "Off", Default {
        n58 = flat-sequence {
          tunnel: w276 -> [w277]
          tunnel: w274 -> [w280]
          tunnel: w275 -> [w279]
          frame #0 {
            n59 = call-poly <vilib>:"WPI_SolenoidSet.vi"("Value"=WPI_SolenoidValue."Forward", "SolenoidDevRef"=w277) -> ()  [unwired: 8 in, 2 out]
          }
          frame #1 {
            w281 = 0.0 ("Output")
            n60 = call <vilib>:"WPI_MotorControlSetOutput.vi"("Output"=w281, "MotorControlDevRef"=w279) -> ()  [unwired: 7 in, 3 out]
            n61 = call <vilib>:"WPI_MotorControlSetOutput.vi"("Output"=w281, "MotorControlDevRef"=w280) -> ()  [unwired: 7 in, 3 out]
          }
        }
      }
      frame "Intake" {
        n62 = flat-sequence {
          tunnel: w282 -> [w285]
          tunnel: w283 -> [w289]
          tunnel: w284 -> [w288]
          frame #0 {
            n63 = call-poly <vilib>:"WPI_SolenoidSet.vi"("Value"=WPI_SolenoidValue."Reverse", "SolenoidDevRef"=w285) -> ()  [unwired: 8 in, 2 out]
          }
          frame #1 {
            n64 = call <vilib>:"WPI_MotorControlSetOutput.vi"("Output"=1.0, "MotorControlDevRef"=w288) -> ()  [unwired: 7 in, 3 out]
            n65 = call <vilib>:"WPI_MotorControlSetOutput.vi"("Output"=-1.0, "MotorControlDevRef"=w289) -> ()  [unwired: 7 in, 3 out]
          }
        }
      }
      frame "Spit Low" {
        n66 = flat-sequence {
          tunnel: w293 -> [w294]
          tunnel: w292 -> [w298]
          tunnel: w291 -> [w297]
          frame #0 {
            n67 = call-poly <vilib>:"WPI_SolenoidSet.vi"("Value"=WPI_SolenoidValue."Reverse", "SolenoidDevRef"=w294) -> ()  [unwired: 8 in, 2 out]
          }
          frame #1 {
            n68 = call <vilib>:"WPI_MotorControlSetOutput.vi"("Output"=0.35, "MotorControlDevRef"=w298) -> ()  [unwired: 7 in, 3 out]
            n69 = call <vilib>:"WPI_MotorControlSetOutput.vi"("Output"=-0.35, "MotorControlDevRef"=w297) -> ()  [unwired: 7 in, 3 out]
          }
        }
      }
      frame "Spit High" {
        n70 = flat-sequence {
          tunnel: w301 -> [w303]
          tunnel: w300 -> [w307]
          tunnel: w302 -> [w306]
          frame #0 {
            n71 = call-poly <vilib>:"WPI_SolenoidSet.vi"("Value"=WPI_SolenoidValue."Reverse", "SolenoidDevRef"=w303) -> ()  [unwired: 8 in, 2 out]
          }
          frame #1 {
            n72 = call <vilib>:"WPI_MotorControlSetOutput.vi"("Output"=0.9, "MotorControlDevRef"=w307) -> ()  [unwired: 7 in, 3 out]
            n73 = call <vilib>:"WPI_MotorControlSetOutput.vi"("Output"=-0.9, "MotorControlDevRef"=w306) -> ()  [unwired: 7 in, 3 out]
          }
        }
      }
    }
    n74 = Greater?(x=w111, y=50.0 ("upper limit")) -> (0:w112:bool)
    n75 = global read "Global Variables.vi" "Elevator Angle"() -> (w123:T24)
    n76 = case shown="\"High\"" w101 {
      tunnel: w128 -> [w219 w220]
      frame "Low", Default {
        n77 = call-poly <vilib>:"WPI_SolenoidSet.vi"("Value"=WPI_SolenoidValue."Forward", "SolenoidDevRef"=w219) -> ()  [unwired: 8 in, 2 out]
      }
      frame "High" {
        n78 = call-poly <vilib>:"WPI_SolenoidSet.vi"("Value"=WPI_SolenoidValue."Reverse", "SolenoidDevRef"=w220) -> ()  [unwired: 8 in, 2 out]
      }
    }
    n79 = Equal?(x=w106, y=enum16{"Low", "High"}."High") -> (x = y?=w104:bool)
    n80 = And(x=w109, y=w112) -> (x .and. y?=w114:bool)
    n81 = case shown="\"Down\"" w140 {
      tunnel: w139 -> [w270 w273]
      frame "Up", Default {
        n82 = call-poly <vilib>:"WPI_SolenoidSet.vi"("Value"=WPI_SolenoidValue."Reverse", "SolenoidDevRef"=w270) -> ()  [unwired: 8 in, 2 out]
      }
      frame "Down" {
        n83 = call-poly <vilib>:"WPI_SolenoidSet.vi"("Value"=WPI_SolenoidValue."Forward", "SolenoidDevRef"=w273) -> ()  [unwired: 8 in, 2 out]
      }
    }
    n84 = case shown="True" w114 {
      tunnel: [w151 w185] -> w92
      tunnel: w111 -> [w156 _]
      tunnel: [w153 TRUE] -> w110
      tunnel: w109 -> [w152 _]
      tunnel: [w149 FALSE] -> w108
      tunnel: w107 -> [w148 _]
      frame False {
        n85 = Greater?(x=w156, y=70.0) -> (0:w154:bool)
        n86 = global read "Global Variables.vi" "Intake Angle Setpoint"() -> (w150:dbl)
        n87 = case shown="True" w154 {
          tunnel: [w170 -170.0 ("Intake Angle Setpoint")] -> w151
          tunnel: [FALSE TRUE] -> w153
          tunnel: w152 -> [_ _]
          tunnel: w150 -> [w178 _]
          tunnel: [w158 FALSE] -> w149
          tunnel: w148 -> [w163 _]
          frame False {
            n88 = Less?(x=w178, y=-140.0) -> (x < y?=w176:bool)
            n89 = global read "Global Variables.vi" "Climb?"() -> (w162:bool)
            n90 = global read "Global Variables.vi" "Elevator Position"() -> (w172:T23)
            n91 = Or(x=w163, y=w162) -> (x .or. y?=w161:bool)
            n92 = Equal?(x=w172, y=T23."Ground") -> (x = y?=w169:bool)
            n93 = Equal?(x=w172, y=T23."Switch") -> (x = y?=w168:bool)
            n94 = Equal?(x=w172, y=T23."Portal") -> (x = y?=w167:bool)
            n95 = Compound Arithmetic op=OR(w169, w168, w167) -> (w160:bool)
            n96 = Not(x=w160) -> (.not. x?=w159:bool)
            n97 = And(x=w161, y=w159) -> (x .and. y?=w158:bool)
            n98 = case shown="True" w158 {
              tunnel: [0.0 -120.0] -> w164
              frame False {
              }
              frame True {
              }
            }
            n99 = global write "Global Variables.vi" "Oh Crap"(FALSE ("Oh Crap")) -> ()
            n100 = Select(t=-120.0, s=w176, f=w164) -> (s? t:f=w166:dbl)
            n101 = Select(t=0.0 ("f"), s=w160, f=w166) -> (s? t:f=w170:dbl)
          }
          frame True {
          }
        }
      }
      frame True {
        n102 = global read "Global Variables.vi" "Oh Crap"() -> (w186:bool)
        n103 = case shown="True" w186 {
          tunnel: [-170.0 ("Intake Angle Setpoint") -130.0 ("Intake Angle Setpoint")] -> w185
          frame False {
          }
          frame True {
          }
        }
      }
    }
    "Elevator Topped Out" <- w110
    n104 = Equal?(x=w101, y=enum16{"Low", "High"}."High") -> (x = y?=w100:bool)
    n105 = case shown="\"Straight Up\"" w123 {
      tunnel: w124 -> [w196 w200 w202 w208 _]
      tunnel: [w196 w199 w204 w207 1.02 ("Linear Actuator Setpoint")] -> w120
      tunnel: [TRUE TRUE TRUE FALSE TRUE] -> w121
      tunnel: w122 -> [_ _ _ w205 _]
      frame "Idle", Default {
      }
      frame "Subtract" {
        n106 = Add(x=0.007, y=w200) -> (x+y=w199:dbl)
      }
      frame "Add" {
        n107 = Subtract(x=w202, y=0.0085 ("x")) -> (x-y=w204:dbl)
      }
      frame "Straight Up" {
        n108 = case shown="True" w205 {
          tunnel: w208 -> [w209 w212]
          tunnel: [w209 w211] -> w207
          frame False {
          }
          frame True {
            n109 = Equal?(x=0.65, y=w212) -> (x = y?=w210:bool)
            n110 = case shown="False" w210 {
              tunnel: [0.65 ("Linear Actuator Setpoint") 1.02 ("Linear Actuator Setpoint")] -> w211
              frame False {
                # "remember to change all"
                # ".65 for comp"
              }
              frame True {
              }
            }
          }
        }
      }
      frame "Portal" {
      }
    }
    n111 = call-poly <vilib>:"NT Write Value.vi"("Boolean"=w104, "Name"="Drive Gear") -> ()  [unwired: 9 in, 1 out]
    n112 = call-poly <vilib>:"NT Write Value.vi"("Boolean"=w100, "Name"="Elevator Gear") -> ()  [unwired: 9 in, 1 out]
    n113 = global read "Global Variables.vi" "Elevator Position"() -> (w129:T23)
    n114 = global read "Global Variables.vi" "Setpoint"() -> (w135:dbl)
    n115 = case shown="\"Ground\"" w129 {
      tunnel: [0.25 ("Setpoint") 25.0 ("Setpoint") 32.0 ("Setpoint") 68.0 ("Setpoint") w241 w250 w261 w265 w267] -> w132
      tunnel: w135 -> [_ _ _ _ w242 w251 w262 w266 w267]
      tunnel: [FALSE ("Cube Up") FALSE ("Cube Up") FALSE ("Cube Up") FALSE ("Cube Up") FALSE ("Cube Up") TRUE ("Cube Up") FALSE ("Cube Up") FALSE ("Cube Up") FALSE ("Cube Up")] -> w134
      tunnel: [FALSE ("Cube Up") FALSE ("Cube Up") FALSE ("Cube Up") FALSE ("Cube Up") TRUE ("Cube Up") FALSE ("Cube Up") FALSE ("Cube Up") FALSE ("Cube Up") FALSE ("Cube Up")] -> w133
      frame "Ground" {
        n116 = global write "Global Variables.vi" "Linear Actuator Setpoint"(0.65 ("Linear Actuator Setpoint")) -> ()
      }
      frame "Portal" {
      }
      frame "Switch" {
        n117 = global write "Global Variables.vi" "Linear Actuator Setpoint"(0.65 ("Linear Actuator Setpoint")) -> ()
      }
      frame "Scale" {
        n118 = global write "Global Variables.vi" "Linear Actuator Setpoint"(0.65 ("Linear Actuator Setpoint")) -> ()
      }
      frame "Cube Down" {
        n119 = case shown="False" "Cube Down" {
          tunnel: w242 -> [w248 w249]
          tunnel: [w247 w249] -> w241
          frame False {
            n120 = Add(x=-11.0, y=w248) -> (x+y=w247:dbl)
          }
          frame True {
          }
        }
      }
      frame "Cube Up" {
        n121 = case shown="False" "Cube Up" {
          tunnel: w251 -> [w257 w258]
          tunnel: [w256 w258] -> w250
          frame False {
            n122 = Add(x=11.0, y=w257) -> (x+y=w256:dbl)
          }
          frame True {
          }
        }
      }
      frame "Add Down" {
        n123 = Decrement(x=w262) -> (x-1=w261:dbl)
        n124 = call "Get Measurements.vi"() -> ()  [unwired: 9 in, 2 out]
      }
      frame "Add Up" {
        n125 = Increment(x=w266) -> (x+1=w265:dbl)
      }
      frame "Idle", Default {
      }
    }
    n126 = call-poly <vilib>:"NT Read Value.vi"("Default Value"=0.0, "Name"="Side") -> ("Numeric"=→"Side":dbl)  [unwired: 8 in, 1 out]
    n127 = call-poly <vilib>:"NT Read Value.vi"("Default Value"=0.0, "Name"="Field Option") -> ("Numeric"=→"Field option":dbl)  [unwired: 8 in, 1 out]
    n128 = local write "Cube Down"(w133) -> ()
    n129 = local write "Cube Up"(w134) -> ()
    n130 = global read "Global Variables.vi" "Climb?"() -> (w115:bool)
    n131 = In Range and Coerce(upper limit=71.0, x=w132, lower limit=0.5) -> (coerced(x)=w119:dbl)  [unwired: 1 out]
    n132 = In Range and Coerce(upper limit=0.92, x=w120, lower limit=0.05) -> (coerced(x)=w117:dbl)  [unwired: 1 out]
    n133 = case shown="True" w115 {
      tunnel: [w191 68.0 ("upper limit")] -> w118
      tunnel: w119 -> [w191 _]
      tunnel: w117 -> [w192 _]
      tunnel: [w192 0.74 ("upper limit")] -> w116
      frame False {
      }
      frame True {
      }
    }
    n134 = global write "Global Variables.vi" "Setpoint"(w118) -> ()
    n135 = global write "Global Variables.vi" "Linear Actuator Setpoint"(w116) -> ()
    n136 = global write "Global Variables.vi" "Intake Angle Setpoint"(w92) -> ()
  }
